vi "Normalize_3.vi"(0 "CursorX":dbl, 1 "Energy Scale in eV":dbl[](array[numeric])=[127.4908344187581, 127.31873082067824, 127.14709125153166, 126.97591383715968, 126.80519671348279, 126.63493802643292, 126.46513593188628, 126.29578859559687, 126.12689419313035, 125.95845090979859, 125.79045694059455, 125.62291049012804, 125.45580977256152, 125.28915301154674, 125.1229384401619, 124.95716430084899, 124.79182884535201, 124.62693033465553, 124.4624670389235, 124.29843723743909, 124.13483921854434, 123.97167127958089, 123.8089317268308, 123.64661887545788, 123.48473104944969, 123.32326658155974, 123.16222381325029, 123.00160109463562, 122.84139678442554, 122.68160924986968, 122.52223686670183, 122.36327801908506, 122.204731099557, 122.0465945089757, 121.88886665646591, 121.7315459593656, 121.57463084317321, 121.41811974149493, 121.26201109599273, 121.10630335633259, 120.95099498013309, 120.79608443291464, 120.64157018804883, 120.48745072670835, 120.33372453781708, 120.18039011800093, 120.02744597153871, 119.87489061031341, 119.72272255376411, 119.57094032883798, 119.41954246994274, 119.2685275188995, 119.11789402489606, 118.96764054444026, 118.81776564131393, 118.66826788652727, 118.51914585827326, 118.37039814188262, 118.22202332977913, 118.07402002143525, 117.92638682332793, 117.77912234889496, 117.63222521849164, 117.48569405934754, 117.33952750552375, 117.19372419787064, 117.04828278398546, 116.90320191817071, 116.75848026139249, 116.61411648123958, 116.47010925188216, 116.3264572540315, 116.18315917489963, 116.04021370815927, 115.89761955390415, 115.75537541860973, 115.6134800150939, 115.47193206247826, 115.33073028614956, 115.18987341772151, 115.04936019499667, 114.90918936192875, 114.76935966858542, 114.62986987111086, 114.49071873168897, 114.35190501850688, 114.2134275057185, 114.07528497340836, 113.93747620755592, 113.8, 113.66285514840335, 113.52604045621774, 113.38955473264906, 113.25339679262285, 113.11756545674993, 112.98205955129238, 112.84687790812978, 112.71201936472555, 112.57748276409363, 112.44326695476556, 112.3093707907574, 112.1757931315372, 112.04253284199272, 111.90958879239916, 111.7769598583872, 111.64464492091145, 111.51264286621885, 111.38095258581748, 111.24957297644548, 111.11850294004033, 110.9877413837082, 110.85728721969349, 110.72713936534886, 110.59729674310515, 110.46775828044161, 110.33852290985651, 110.20958956883761, 110.08095719983332, 109.95262475022349, 109.82459117229091, 109.69685542319272, 109.56941646493202, 109.44227326432996, 109.31542479299759, 109.18887002730828, 109.06260794837013, 108.93663754199864, 108.81095779868954, 108.68556771359184, 108.56046628648103, 108.43565252173258, 108.3111254282953, 108.1868840196654, 108.0629273138602, 107.93925433339238, 107.8158641052443, 107.69275566084237, 107.56992803603184, 107.44738027105151, 107.32511141050885, 107.20312050335508, 107.08140660286051, 106.95996876659015, 106.83880605637928, 106.71791753830934, 106.59730228268388, 106.47695936400481, 106.35688786094873, 106.23708685634325, 106.11755543714389, 105.99829269441072, 105.87929772328529, 105.7605696229679, 105.64210749669479, 105.52391045171547, 105.4059775992704, 105.28830805456877, 105.17090093676624, 105.053755368943, 104.93687047808199, 104.82024539504715, 104.70387925456193, 104.5877711951878, 104.47192035930317, 104.35632589308207, 104.24098694647329, 104.12590267317951, 104.01107223063666, 103.89649477999322, 103.78216948608994, 103.66809551743951, 103.55427204620634, 103.44069824818654, 103.32737330278816, 103.21429639301127, 103.10146670542836, 102.98888343016489, 102.87654576087992, 102.76445289474677, 102.65260403243391, 102.54099837808613, 102.42963513930542, 102.3185135271323, 102.20763275602735, 102.09699204385247, 101.98659061185258, 101.87642768463736, 101.76650249016316, 101.65681425971482, 101.5473622278878, 101.43814563257054, 101.32916371492648, 101.22041571937669, 101.11190089358244, 101.00361848842766, 100.89556775800186, 100.78774795958289, 100.68015835362012, 100.57279820371727, 100.46566677661575, 100.35876334217804, 100.25208717337092, 100.1456375462491, 100.03941373993885, 99.93341503662172, 99.82764072151829, 99.72209008287223, 99.61676241193423, 99.51165700294621, 99.40677315312547, 99.30211016264917, 99.19766733463862, 99.09344397514386, 98.98943939312832, 98.88565290045356, 98.782083811864, 98.67873144497192, 98.57559512024245, 98.47267416097874, 98.36996789330698, 98.26747564616193, 98.1651967512721, 98.06313054314539, 97.96127635905448, 97.8596335390227, 97.75820142580957, 97.65697936489674, 97.55596670447393, 97.4551627954249, 97.3545669913135, 97.25417864836994, 97.15399712547705, 97.05402178415653, 96.9542519885555, 96.85468710543297, 96.75532650414647, 96.65616955663866, 96.55721563742419, 96.45846412357652, 96.35991439471479, 96.26156583299094, 96.16341782307668, 96.06546975215075, 95.96772100988608, 95.87017098843721, 95.77281908242763, 95.67566468893722, 95.5787072074899, 95.48194604004124, 95.38538059096602, 95.28901026704625, 95.19283447745882, 95.09685263376352, 95.00106414989101, 94.90546844213091, 94.81006492911996, 94.71485303183015, 94.61983217355709, 94.5250017799084, 94.43036127879196, 94.33591010040465, 94.24164767722067, 94.14757344398038, 94.05368683767887, 93.95998729755478, 93.8664742650791, 93.77314718394416, 93.68000550005246, 93.58704866150585, 93.49427611859448, 93.40168732378613, 93.30928173171532, 93.21705879917258, 93.12501798509395, 93.03315875055024, 92.94148055873663, 92.84998287496211, 92.75866516663919, 92.66752690327348, 92.57656755645348, 92.48578659984031, 92.3951835091576, 92.30475776218141, 92.21450883873013, 92.12443622065456, 92.03453939182799, 91.94481783813634, 91.85527104746834, 91.76589850970578, 91.67669971671388, 91.58767416233158, 91.49882134236205, 91.41014075456309, 91.32163189863773, 91.23329427622478, 91.14512739088953, 91.05713074811436, 90.9693038552896, 90.88164622170424, 90.79415735853689, 90.70683677884657, 90.61968399756383, 90.53269853148161, 90.44587989924644, 90.35922762134948, 90.27274122011771, 90.18642021970518, 90.10026414608427, 90.01427252703695, 89.9284448921463, 89.84278077278776, 89.75727970212071, 89.67194121508, 89.5867648483674, 89.50175014044336, 89.4168966315186, 89.33220386354577, 89.24767138021139, 89.16329872692738, 89.0790854508232, 88.9950311007375, 88.91113522721028, 88.82739738247469, 88.74381712044917, 88.66039399672954, 88.57712756858102, 88.49401739493054, 88.41106303635885, 88.32826405509279, 88.24562001499761, 88.16313048156933, 88.08079502192706, 87.99861320480551, 87.9165846005474, 87.834708781096, 87.75298531998766, 87.67141379234444, 87.5899937748667, 87.50872484582584, 87.42760658505698, 87.34663857395171, 87.26582039545089, 87.18515163403755, 87.10463187572967, 87.02426070807317, 86.94403772013486, 86.86396250249541, 86.7840346472424, 86.70425374796338, 86.62461939973902, 86.5451311991362, 86.46578874420126, 86.3865916344532, 86.30753947087689, 86.22863185591646, 86.14986839346858, 86.07124868887585, 85.99277234892017, 85.91443898181625, 85.83624819720504, 85.75819960614727, 85.68029282111699, 85.60252745599519, 85.52490312606331, 85.44741944799702, 85.37007603985991, 85.29287252109714, 85.21580851252916, 85.13888363634568, 85.06209751609936, 84.98544977669961, 84.90894004440669, 84.83256794682544, 84.75633311289931, 84.68023517290442, 84.60427375844343, 84.52844850243974, 84.45275903913151, 84.37720500406576, 84.30178603409257, 84.22650176735924, 84.15135184330448, 84.07633590265272, 84.00145358740829, 83.92670454084981, 83.85208840752448, 83.77760483324245, 83.70325346507123, 83.62903395133011, 83.55494594158463, 83.48098908664102, 83.40716303854072, 83.33346745055499, 83.25990197717947, 83.18646627412863, 83.11315999833063, 83.03998280792182, 82.96693436224146, 82.89401432182646, 82.82122234840608, 82.74855810489677, 82.67602125539688, 82.60361146518153, 82.53132840069749, 82.459171729558, 82.38714112053766, 82.3152362435675, 82.24345676972975, 82.17180237125297, 82.10027272150694, 82.02886749499785, 81.95758636736322, 81.88642901536704, 81.81539511689493, 81.7444843509492, 81.67369639764406, 81.60303093820082, 81.53248765494305, 81.46206623129191, 81.39176635176132, 81.32158770195329, 81.25152996855326, 81.18159283932538, 81.11177600310793, 81.04207914980866, 80.9725019704002, 80.90304415691556, 80.83370540244348, 80.76448540112398, 80.69538384814386, 80.62640043973224, 80.55753487315599, 80.48878684671548, 80.42015605974007, 80.3516422125837, 80.28324500662062, 80.214964144241, 80.1467993288466, 80.07875026484648, 80.01081665765278, 79.94299821367642, 79.87529464032283, 79.80770564598788, 79.74023094005352, 79.67287023288377, 79.60562323582045, 79.53848966117914, 79.47146922224508, 79.40456163326897, 79.33776660946309, 79.27108386699715, 79.20451312299421, 79.13805409552688, 79.07170650361311, 79.0054700672124, 78.93934450722176, 78.87332954547185, 78.80742490472305, 78.74163030866158, 78.67594548189567, 78.61037014995165, 78.54490403927016, 78.47954687720245, 78.41429839200637, 78.34915831284282, 78.28412636977188, 78.21920229374913, 78.15438581662194, 78.08967667112572, 78.02507459088032, 77.96057931038636, 77.89619056502156, 77.83190809103714, 77.7677316255542, 77.70366090656022, 77.63969567290535, 77.57583566429899, 77.5120806213062, 77.44843028534419, 77.38488439867884, 77.3214427044212, 77.25810494652407, 77.19487086977846, 77.13174021981034, 77.068712743077, 77.00578818686385, 76.94296629928093, 76.8802468292596, 76.81762952654918, 76.75511414171359, 76.69270042612816, 76.63038813197612, 76.56817701224551, 76.50606682072588, 76.44405731200496, 76.38214824146549, 76.32033936528197, 76.25863044041756, 76.19702122462074, 76.13551147642222, 76.07410095513187, 76.01278942083536, 75.95157663439127, 75.89046235742782, 75.82944635233987, 75.76852838228581, 75.70770821118442, 75.646985603712, 75.58636032529915, 75.52583214212783, 75.46540082112838, 75.40506612997649, 75.34482783709021, 75.28468571162703, 75.22463952348092, 75.16468904327932, 75.10483404238036, 75.04507429286986, 74.9854095675584, 74.92583963997858, 74.866364284382, 74.80698327573653, 74.74769638972337, 74.6885034027343, 74.62940409186886, 74.57039823493153, 74.51148561042892, 74.45266599756708, 74.39393917624865, 74.33530492707015, 74.27676303131935, 74.2183132709723, 74.15995542869092, 74.10168928782007, 74.04351463238501, 73.98543124708868, 73.92743891730902, 73.86953742909643, 73.81172656917096, 73.75400612491987, 73.69637588439493, 73.63883563630985, 73.58138517003768, 73.52402427560823, 73.46675274370561, 73.40957036566554, 73.35247693347291, 73.29547223975923, 73.23855607780014, 73.18172824151284, 73.12498852545372, 73.06833672481577, 73.0117726354262, 72.95529605374392, 72.89890677685717, 72.84260460248103, 72.786389328955, 72.73026075524066, 72.67421868091921, 72.61826290618909, 72.5623932318636, 72.50660945936862, 72.45091139074016, 72.39529882862199, 72.33977157626349, 72.2843294375171, 72.22897221683617, 72.1736997192726, 72.1185117504746, 72.0634081166843, 72.00838862473559, 71.95345308205187, 71.89860129664369, 71.84383307710664, 71.78914823261907, 71.73454657293985, 71.68002790840616, 71.62559204993138, 71.57123880900284, 71.51696799767959, 71.46277942859035, 71.40867291493129, 71.35464827046387, 71.30070530951272, 71.24684384696356, 71.19306369826097, 71.13936467940643, 71.08574660695604, 71.03220929801866, 70.9787525702536, 70.92537624186869, 70.8720801316182, 70.81886405880076, 70.7657278432573, 70.7126713053691, 70.65969426605567, 70.6067965467728, 70.5539779695105, 70.50123835679108, 70.4485775316671, 70.39599531771938, 70.34349153905511, 70.29106602030579, 70.23871858662535, 70.18644906368817, 70.13425727768717, 70.08214305533185, 70.03010622384639, 69.97814661096777, 69.92626404494382, 69.87445835453133, 69.82272936899422, 69.77107691810161, 69.71950083212599, 69.66800094184129, 69.61657707852116, 69.56522907393699, 69.51395676035614, 69.46275997054013, 69.4116385377428, 69.36059229570847, 69.3096210786702, 69.25872472134796, 69.20790305894681, 69.15715592715519, 69.1064831621431, 69.0558846005604, 69.00536007953494, 68.95490943667092, 68.9045325100471, 68.8542291382151, 68.8039991601976, 68.75384241548677, 68.70375874404237, 68.65374798629018, 68.60380998312033, 68.55394457588544, 68.50415160639912, 68.45443091693427, 68.40478235022128, 68.35520574944653, 68.30570095825065, 68.25626782072695, 68.20690618141965, 68.15761588532239, 68.10839677787658, 68.05924870496968, 68.01017151293372, 67.96116504854368, 67.9122291590158, 67.86336369200605, 67.8145684956086, 67.7658434183542, 67.71718830920857, 67.6686030175709, 67.62008739327233, 67.57164128657428, 67.523264548167, 67.47495702916804, 67.42671858112067, 67.37854905599242, 67.3304483061735, 67.28241618447537, 67.23445254412914, 67.18655723878418, 67.13873012250656, 67.0909710497776, 67.04327987549235, 66.9956564549582, 66.94810064389335], 2 "raw data":dbl[](array[numeric]), 3 "Normalize":bool) -> (6 "Counts at X":dbl, 7 "raw data":dbl[](array[numeric]), 9 "Max. Wert":dbl)   [LabVIEW 2013]
panel:
  # "Wenn man diese Bezugsskala (hier Energy Scale) nicht angibt,\ndann liest der Cursor nicht den richtigen Wert aus!"
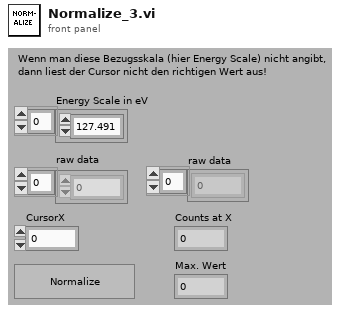
[diagram p1: front panel]
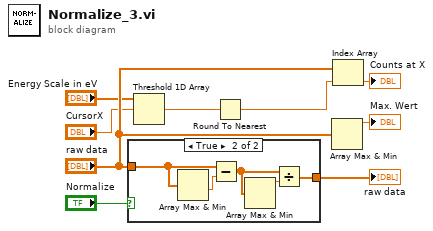
[diagram p0: block diagram]
diagram:
  n1 = case shown="True" "Normalize" {
    tunnel: [w10 w12] -> w6
    tunnel: "raw data" -> [w10 w11]
    frame False {
    }
    frame True {
      n2 = Array Max & Min(array=w11) -> (min value=w15:dbl)  [unwired: 3 out]
      n3 = Subtract(x=w11, y=w15) -> (x-y=w14:dbl[])
      n4 = Array Max & Min(array=w14) -> (max value=w13:dbl)  [unwired: 3 out]
      n5 = Divide(x=w14, y=w13) -> (x/y=w12:dbl[])
    }
  }
  "raw data" <- w6
  n6 = Threshold 1D Array(2:"CursorX", 3:"Energy Scale in eV") -> (0:w2:dbl)  [unwired: 1 in]
  n7 = Round To Nearest(number=w2) -> (nearest integer value=w1:dbl)
  n8 = Array Max & Min(array="raw data") -> (max value=→"Max. Wert":dbl)  [unwired: 3 out]
  n9 = Index Array(array="raw data", index=w1) -> (element=→"Counts at X":dbl)
